vi "f2c.vi"() -> ()   [LabVIEW 2009]
panel:
  in  "Numeric 2":dbl
  in  "Numeric":dbl
  in  "Slide":dbl(slide) scale=0.0..100.0
  out "Thermometer":dbl(slide) scale=0.0..100.0
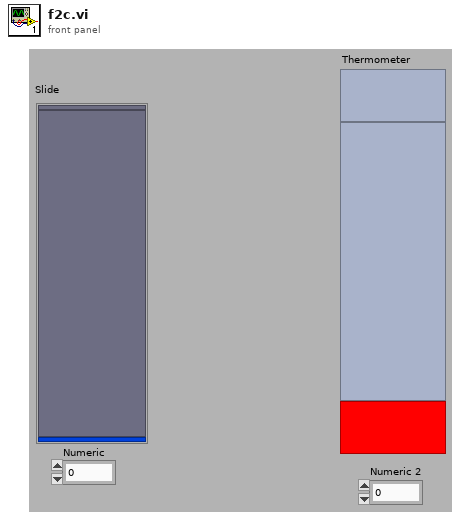
[diagram p1: front panel]
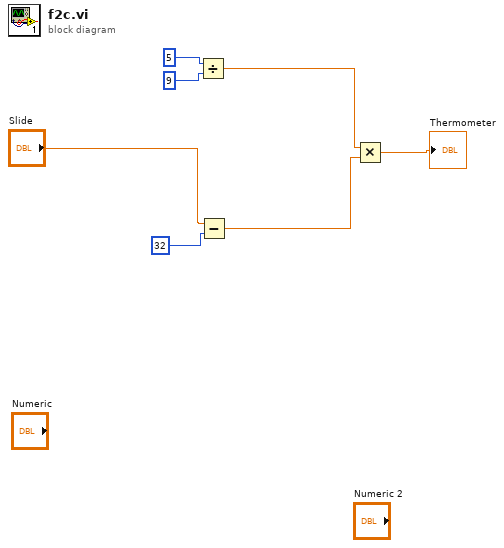
[diagram p0: block diagram]
diagram:
  n1 = Divide(x=5, y=9) -> (x/y=w3:dbl)
  n2 = Subtract(x="Slide", y=32) -> (x-y=w4:dbl)
  n3 = Multiply(x=w3, y=w4) -> (x*y=→"Thermometer":dbl)
